vi "writeToXML.vi"(8 "error in (no error)":errorcluster, 10 "ClassLabel":string, 11 "ScienceTargetConfiguration in":refnum<class "ScienceTargetConfiguration.lvclass">) -> (0 "error out":errorcluster, 2 "XML out":string, 3 "ScienceTargetConfiguration out":refnum<class "ScienceTargetConfiguration.lvclass">)   [LabVIEW 2022 SP3, in "TCSDataDefinitions.lvlib" / "TCSCommand.lvlib" / "TargetConfiguration.lvlib" / "ScienceTargetConfiguration.lvclass"]
uses:
  ScienceTargetConfiguration.lvclass
  ScienceTargetConfiguration.lvclass/ScienceTargetConfiguration.ctl
  TargetConfiguration/TargetConfiguration.lvclass
  Rotator/Rotator.lvclass
  <userlib>/Common/XML/XMLGenerator/XMLGenerator.lvclass
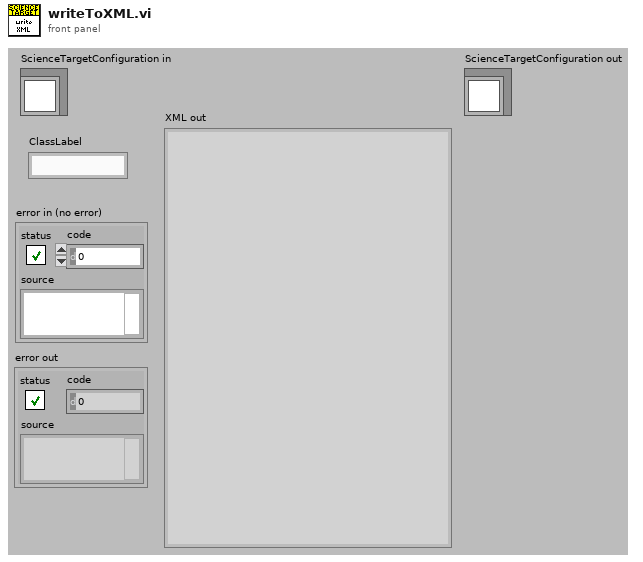
[diagram p1: front panel]
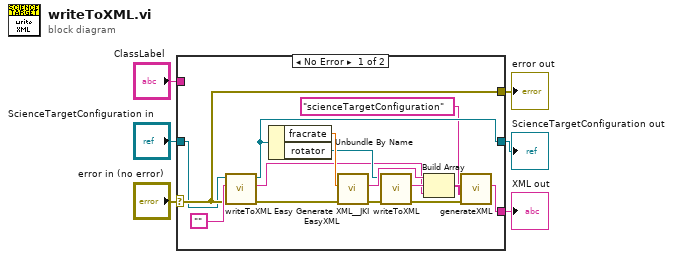
[diagram p0: block diagram]
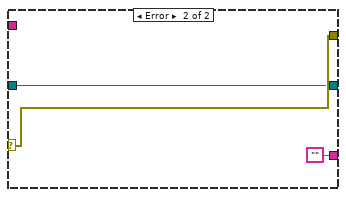
[diagram p2: hidden frame]
diagram:
  n1 = case shown="No Error" "error in (no error)" {
    selector: "error in (no error)" -> [w20 w24]
    tunnel: [w20 w24] -> w5
    tunnel: [w15 w23] -> w3
    tunnel: "ScienceTargetConfiguration in" -> [w16 w23]
    tunnel: [w10 ""] -> w2
    tunnel: "ClassLabel" -> [_ _]
    frame No Error {
      n2 = call-parent "writeToXML.vi"("error in (no error)"=w20, "classLabel"="", "TargetConfiguration in"=w16) -> ("error out"=w17:errorcluster, "XML out"=w7:string, "TargetConfiguration out"=w15:refnum<class "ScienceTargetConfiguration.lvclass">)  [unwired: 6 in]
      n3 = Unbundle By Name(w15) -> ("fracrate"=w19:dbl, "rotator"=w14:refnum<class "Rotator.lvclass">)
      n4 = call <vilib>:"Easy Generate XML__JKI EasyXML.vi"("error in (no error)"=w17, "LabVIEW Data"=w19) -> ("error out"=w9:errorcluster, "XML String"=w18:string)  [unwired: 8 in]
      n5 = call-dynamic "writeToXML.vi"("error in (no error)"=w9, "Rotator in"=w14) -> ("error out"=w8:errorcluster, "XML out"=w13:string)  [unwired: 7 in, 1 out]
      n6 = Build Array(w18, w13, w7) -> (w12:string[])
      n7 = call <userlib>:"generateXML.vi"("error in"=w8, "childrenXML"=w12, "elementName"="scienceTargetConfiguration" ("Class Label")) -> ("XML out"=w10:string)  [unwired: 6 in, 2 out]
    }
    frame Error {
    }
  }
  "error out" <- w5
  "ScienceTargetConfiguration out" <- w3
  "XML out" <- w2
